vi "Shooter Limit.vi"(1 "Check?":bool, 2 "Enum":enum16{"Start", "Run", "End"}(ring)) -> (0 "Value":bool)   [LabVIEW 2014]
uses:
  TypeDefs/Digital Module 1.ctl
  <vilib>/Rock Robotics/SystemInterfaces/Typedef/FPGA_TypedefDigitalModule.ctl
  <vilib>/Rock Robotics/SystemInterfaces/DIO/FPGA_DIOChannel.ctl
panel:
  in  "Digital Module A":T1={"Module"=enum."Digital Module 1", "L Encoder A"=enum."DIO 1", "L Encoder B"=enum."DIO 2", "R Encoder A"=enum."DIO 3", "R Encoder B"=enum."DIO 4", "Compressor"=enum."DIO 5", "Shooter Limit"=enum."DIO 6", "LED 1"=enum."DIO 7", "LED 2"=enum."DIO 8", "LED 3"=enum."DIO 9", "LED 4"=enum."DIO 9", "Shooter Limit 2"=enum."DIO 11", "Unassigned"=enum."DIO 12", "Unassigned"=enum."DIO 13", "Unassigned"=enum."DIO 14"}
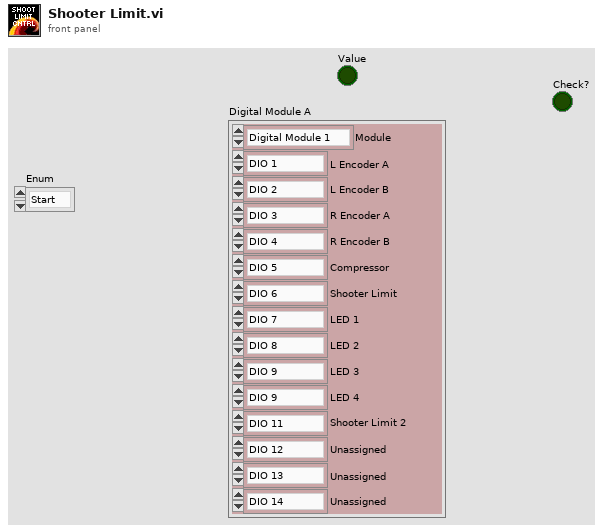
[diagram p1: front panel]
types:
  T1 = typedef "Digital Module 1.ctl" = cluster{"Module":T2, "L Encoder A":T3, "L Encoder B":T3, "R Encoder A":T3, "R Encoder B":T3, "Compressor":T3, "Shooter Limit":T3, "LED 1":T3, "LED 2":T3, "LED 3":T3, "LED 4":T3, "Shooter Limit 2":T3, "Unassigned":T3, "Unassigned":T3, "Unassigned":T3}
  T2 = typedef "FPGA_TypedefDigitalModule.ctl" = enum16{"Digital Module 1", "Digital Module 2"}
  T3 = typedef "FPGA_DIOChannel.ctl" = enum8{"DIO 1", "DIO 2", "DIO 3", "DIO 4", "DIO 5", "DIO 6", "DIO 7", "DIO 8", "DIO 9", "DIO 10", "DIO 11", "DIO 12", "DIO 13", "DIO 14", "Invalid"}
  T4 = typedef "WPI_DigitalInputDevRef.ctl" = cluster{"DevStatus":errorcluster, "DIO Channel":T3, "Digital Module":T2}
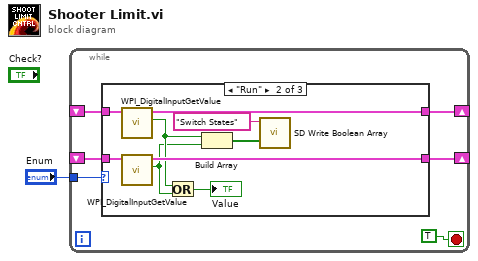
[diagram p0: block diagram]
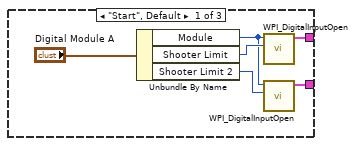
[diagram p2: hidden frame]
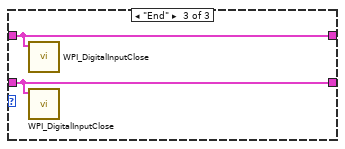
[diagram p3: hidden frame]
diagram:
  n1 = while {
    tunnel: "Enum" -> [w6]
    shift-right: [w4] -> _
    shift-left: _ -> [w5]
    shift-right: [w3] -> _
    shift-left: _ -> [w2]
    stop <- TRUE stop-if-true
    n2 = case shown="\"Run\"" w6 {
      tunnel: w5 -> [_ w22 w24]
      tunnel: [w11 w21 w24] -> w4
      tunnel: [w10 w18 w23] -> w3
      tunnel: w2 -> [_ w20 w23]
      frame "Start", Default {
        n3 = Unbundle By Name("Digital Module A") -> ("Module"=w9:T2, "Shooter Limit"=w12:T3, "Shooter Limit 2"=w8:T3)
        n4 = call <vilib>:"WPI_DigitalInputOpen.vi"("DIO Channel"=w12, "Digital Module (Module 1)"=w9) -> ("DigitalInputDevRef"=w11:T4)  [unwired: 8 in, 1 out]
        n5 = call <vilib>:"WPI_DigitalInputOpen.vi"("DIO Channel"=w8, "Digital Module (Module 1)"=w9) -> ("DigitalInputDevRef"=w10:T4)  [unwired: 8 in, 1 out]
      }
      frame "Run" {
        n6 = call <vilib>:"WPI_DigitalInputGetValue.vi"("DigitalInputDevRef"=w22) -> ("Value"=w17:bool, "DigitalInputDevRef"=w21:T4)  [unwired: 8 in, 1 out]
        n7 = call <vilib>:"WPI_DigitalInputGetValue.vi"("DigitalInputDevRef"=w20) -> ("Value"=w16:bool, "DigitalInputDevRef"=w18:T4)  [unwired: 8 in, 1 out]
        n8 = Or(x=w17, y=w16) -> (x .or. y?=→"Value":bool)
        n9 = Build Array(w17, w16) -> (w15:bool[])
        n10 = call <vilib>:"SD Write Boolean Array.vi"("Boolean Array"=w15, "Name"="Switch States") -> ()  [unwired: 8 in, 2 out]
      }
      frame "End" {
        n11 = call <vilib>:"WPI_DigitalInputClose.vi"("DigitalInputDevRef"=w24) -> ()  [unwired: 10 in, 1 out]
        n12 = call <vilib>:"WPI_DigitalInputClose.vi"("DigitalInputDevRef"=w23) -> ()  [unwired: 10 in, 1 out]
      }
    }
  }
